vi "Read Meta Value.vi"(8 "error in (no error)":errorcluster, 10 "Meta Name":string, 11 "VolatusConfigElement in":refnum<class "VolatusConfigElement.lvclass">) -> (0 "error out":errorcluster, 2 "Meta Value":string, 3 "VolatusConfigElement out":refnum<class "VolatusConfigElement.lvclass">)   [LabVIEW 2020, in "VolatusConfig.lvlib" / "VolatusConfigElement.lvclass"]
uses:
  VolatusConfigElement.lvclass
  VolatusConfigElement.lvclass/VolatusConfigElement.ctl
  lv-cdm/CDM-Config/Config Element/Config Element.lvclass
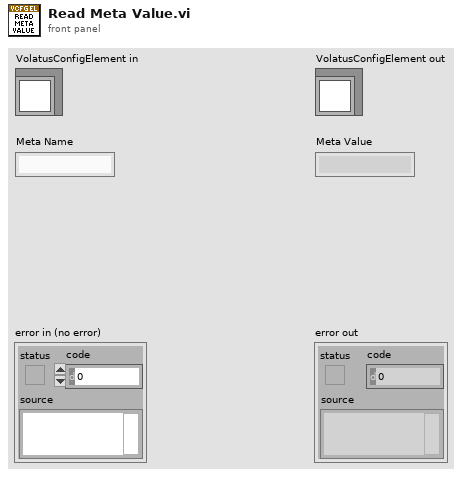
[diagram p1: front panel]
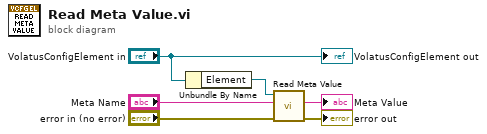
[diagram p0: block diagram]
diagram:
  n1 = Unbundle By Name("VolatusConfigElement in") -> ("Element"=w5:refnum<class "Config Element.lvclass">)
  n2 = call "Read Meta Value.vi"("error in (no error)"="error in (no error)", "Meta Name"="Meta Name", "Config Element in"=w5) -> ("error out"=→"error out":errorcluster, "Meta Value"=→"Meta Value":string)  [unwired: 6 in, 1 out]
  "VolatusConfigElement out" <- "VolatusConfigElement in"
